vi "fix custom device xml.vi"(8 "error in (no error)":errorcluster, 10 "new xml path":path, 11 "NIVS_CDW_MetaDataObj in":refnum<class "NIVS_ScriptedModuleTemplate_MetaDataObj.lvclass">) -> (0 "error out":errorcluster)   [LabVIEW 2014, in "NIVS_ScriptedModuleTemplate_MetaDataObj.lvclass"]
uses:
  NIVS_ScriptedModuleTemplate_MetaDataObj.lvclass
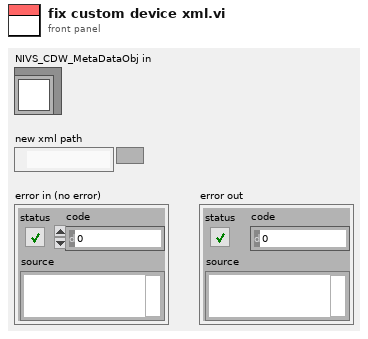
[diagram p1: front panel]
types:
  T1 = enum16{"open", "replace", "create", "open or create", "replace or create", "replace or create with confirmation"}
  T2 = typedef "CD Wizard - Extra Page Name and GUID.ctl" = cluster{"Page Name":string, "Page GUID":string}
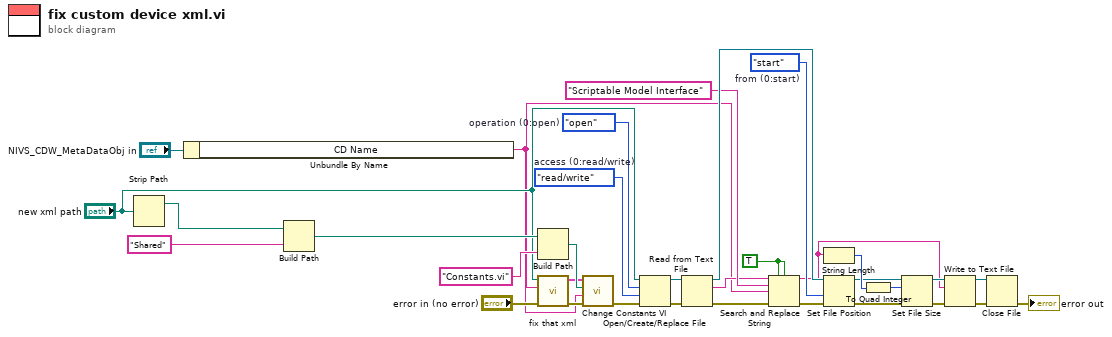
[diagram p0: block diagram]
diagram:
  w29 = enum16{"start", "end", "current"}."start"  # from (0:start)
  w22 = TRUE ("replace all? (F)")
  w17 = T1."open"  # operation (0:open)
  w16 = enum16{"read/write", "read-only", "write-only"}."read/write"  # access (0:read/write)
  n1 = Strip Path(path="new xml path") -> (stripped path=w11:path)  [unwired: 1 out]
  n2 = Unbundle By Name("NIVS_CDW_MetaDataObj in") -> ("CD Name"=w1:string)
  n3 = Build Path(base path=w11, name or relative path="Shared") -> (appended path=w10:path)
  n4 = Build Path(base path=w10, name or relative path="Constants.vi") -> (appended path=w7:path)
  n5 = call "fix that xml.vi"("error in (no error)"="error in (no error)", "nw CD name"=w1, "Path"="new xml path") -> ("error out"=w12:errorcluster, "Extra Pages"=w6:T2[])  [unwired: 7 in]
  n6 = call "Change Constants VI.vi"("error in (no error)"=w12, "new cd name"=w1, "Constants.vi path"=w7, "Extra Pages"=w6) -> ("error out"=w5:errorcluster)  [unwired: 7 in]
  n7 = Open/Create/Replace File(file path (use dialog)="new xml path", error in=w5, operation (0:open)=w17, access (0:read/write)=w16) -> (refnum out=w14:refnum<file>, error out=w15:errorcluster)  [unwired: 3 out]
  n8 = Read from Text File(file (use dialog)=w14, error in=w15) -> (refnum out=w32:refnum<file>, text=w19:string, error out=w20:errorcluster)  [unwired: 3 out]
  n9 = Search and Replace String(replace all?=w22, case sensitive?=w22, input string=w19, search string="Scriptable Model Interface", replace string=w1, error in=w20) -> (result string=w13:string, error out=w33:errorcluster)  [unwired: 2 in, 2 out]
  n10 = String Length(string=w13) -> (length=w30:i32)
  n11 = Set File Position(refnum=w32, from (0:start)=w29, error in=w33) -> (refnum out=w28:refnum<file>, error out=w27:errorcluster)  [unwired: 1 out]
  n12 = To Quad Integer(1:w30) -> (0:w31:i64)
  n13 = Set File Size(4:w27, 6:w31, 7:w28) -> (0:w25:errorcluster, 3:w26:refnum<file>)
  n14 = Write to Text File(file (use dialog)=w26, text=w13, error in=w25) -> (refnum out=w23:refnum<file>, error out=w24:errorcluster)  [unwired: 2 out]
  n15 = Close File(refnum=w23, error in=w24) -> (error out=→"error out":errorcluster)  [unwired: 1 out]
